vi "File Not Found Error Core.vi"(7 "Custom Message":string, 8 "error in":errorcluster, 11 "path in":path) -> (0 "error out":errorcluster)   [LabVIEW 2021, in "File_CIF_U.lvlib"]
uses:
  File_CIF_U.lvlib
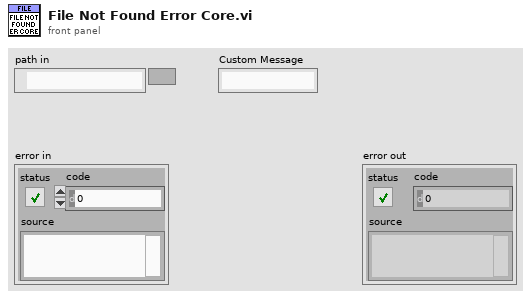
[diagram p1: front panel]
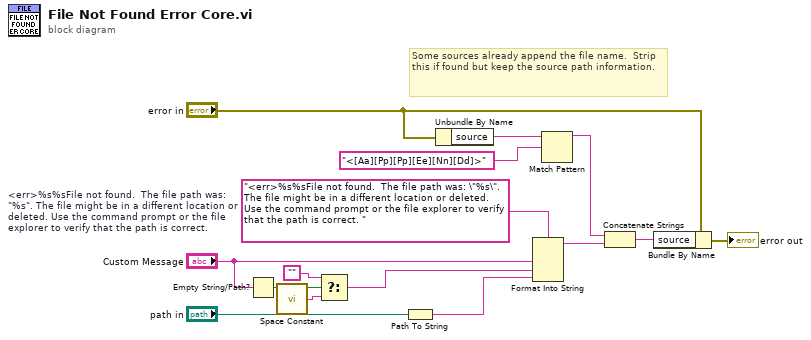
[diagram p0: block diagram]
diagram:
  w13 = "<err>%s%sFile not found.  The file path was: \"%s\". The file might be in a different location or deleted. Use the command prompt or the file explorer to verify that the path is correct. "  # <err>%s%sFile not found.  The file path was: "%s". The file might be in a different location or deleted. Use the command prompt or the file explorer to verify that the path is correct.
  # "Some sources already append the file name.  Strip this if found but keep the source path information."
  n1 = Empty String/Path?(string/path="Custom Message") -> (empty?=w5:bool)
  n2 = call <vilib>:"Space Constant.vi"() -> ("String"=w3:string)
  n3 = Select(t="", s=w5, f=w3) -> (s? t:f=w2:string)
  n4 = Path To String(path="path in") -> (string=w7:string)
  n5 = Unbundle By Name("error in") -> ("source"=w10:string)
  n6 = Format Into String(format string=w13, "Custom Message", w2, w7) -> (resulting string=w1:string)  [unwired: 2 in, 1 out]
  n7 = Match Pattern(string=w10, regular expression="<[Aa][Pp][Pp][Ee][Nn][Dd]>" ("don't translate!")) -> (before substring=w9:string)  [unwired: 1 in, 3 out]
  n8 = Concatenate Strings(w9, w1) -> (w12:string)
  n9 = Bundle By Name(cluster="error in", "source"=w12) -> (→"error out":errorcluster)
